vi "TrajGenAverage.vi"(6 "Init":bool, 8 "error in (no error)":errorcluster, 10 "Ankle Traj Last Step":dbl[][](array[numeric]), 11 "ForceField in":refnum<class "ForceField.lvclass">) -> (0 "error out":errorcluster, 1 "Good Traj":bool, 2 "Ankle Traj Averaged":dbl[][](array[numeric]), 3 "ForceField out":refnum<class "ForceField.lvclass">)   [LabVIEW 2016, in "ForceField.lvclass"]
uses:
  ForceField.lvclass
  ForceField.lvclass/ForceField.ctl
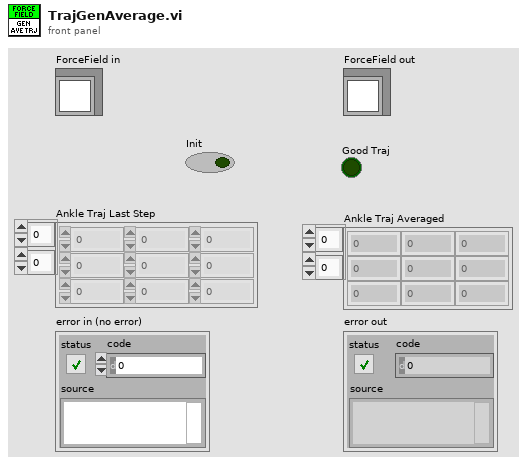
[diagram p1: front panel]
types:
  T1 = typedef "ForceField.lvclass/AnkleTrajPt.ctl" = cluster{"P1":dbl[], "P2":dbl[], "P1-P2":dbl[], "(P1-P2)^2":dbl}
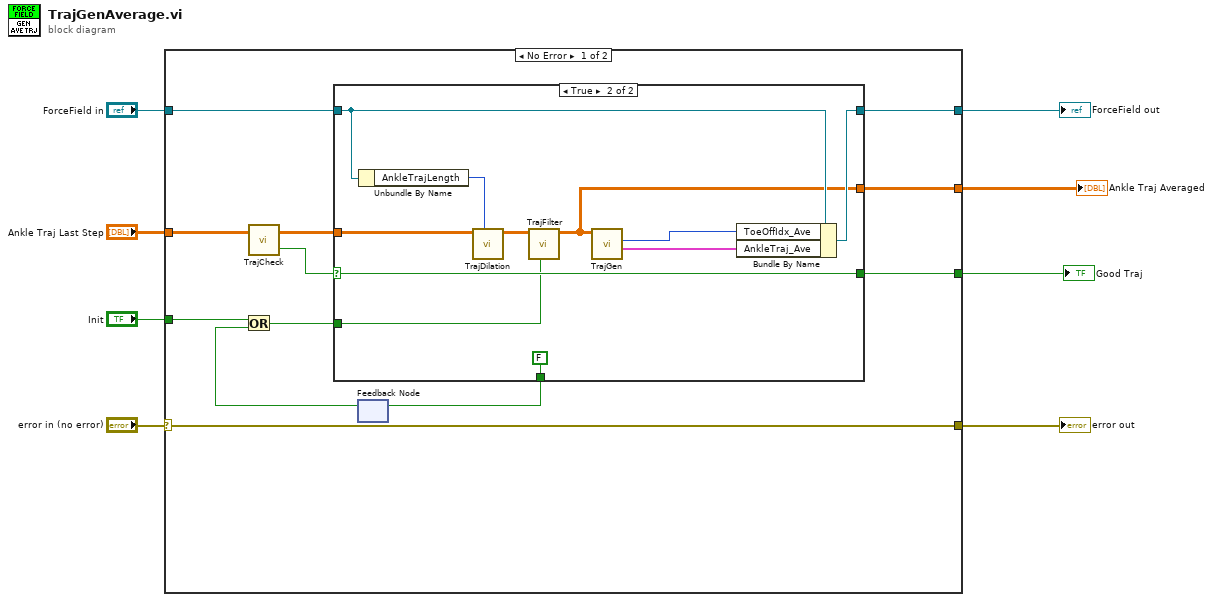
[diagram p0: block diagram]
diagram:
  n1 = case shown="No Error" "error in (no error)" {
    selector: "error in (no error)" -> [w18 w36]
    tunnel: [w18 w36] -> w7
    tunnel: "ForceField in" -> [w20 w35]
    tunnel: [w19 w35] -> w5
    tunnel: "Ankle Traj Last Step" -> [w16 _]
    tunnel: "Init" -> [w9 _]
    tunnel: [w17 _] -> w2
    tunnel: [w14 _] -> w1
    frame No Error {
      n2 = call "TrajCheck.vi"("Traj In"=w16) -> ("Good Trajectory?"=w15:bool, "Traj dup"=w13:dbl[][])  [unwired: 1 in]
      n3 = feedback #1() -> (w11:bool)  [unwired: 1 in]
      n4 = Or(x=w9, y=w11) -> (x .or. y?=w10:bool)
      n5 = case shown="True" w15 {
        selector: w15 -> [w22 w26]
        tunnel: w20 -> [w23 w32]
        tunnel: [w23 w31] -> w19
        tunnel: [_ w28] -> w17
        tunnel: w13 -> [_ w27]
        tunnel: [w22 w26] -> w14
        tunnel: [w21 FALSE] -> w12
        tunnel: w10 -> [w21 w25]
        frame False {
        }
        frame True {
          n6 = Unbundle By Name(w32) -> ("AnkleTrajLength"=w33:i32)
          n7 = call "TrajDilation.vi"("Length"=w33, "TrajBeforeDilation"=w27) -> ("TrajAfterDilation"=w34:dbl[][])  [unwired: 9 in]
          n8 = call "TrajFilter.vi"("Init"=w25, "Traj of Last Step"=w34) -> ("Averaged Traj"=w28:dbl[][])  [unwired: 7 in]
          n9 = call "TrajGen.vi"("AnkleTraj"=w28) -> ("AnkleTraj"=w29:T1[], "ToeOffIdx"=w30:i32)  [unwired: 5 in, 2 out]
          n10 = Bundle By Name(cluster=w32, "ToeOffIdx_Ave"=w30, "AnkleTraj_Ave"=w29) -> (w31:refnum<class "ForceField.lvclass">)
        }
      }
      n11 = feedback-in #1(w12) -> ()
    }
    frame Error {
    }
  }
  "error out" <- w7
  "ForceField out" <- w5
  "Ankle Traj Averaged" <- w2
  "Good Traj" <- w1
